vi "test_Read Digital Static In.vi"(8 "error in (no error)":errorcluster, 11 "TestCase in":refnum<class "FPGA Addon Speciality IO Tests.lvclass">) -> (0 "error out":errorcluster, 3 "TestCase out":refnum<class "FPGA Addon Speciality IO Tests.lvclass">)   [LabVIEW 2020, in "FPGA Addon Speciality IO Tests.lvclass"]
uses:
  FPGA Addon Speciality IO Tests.lvclass
  C:/Users/Administrator/Desktop/GIT/niveristand-custom-device-testing-tools/VeriStandTestCase/VeriStandTestCase.lvclass
  <vilib>/addons/_JKI Toolkits/VI Tester/TestCase.llb/TestCase.lvclass
  FPGA Addon Test Class/FPGA Addon Test Class.lvclass
  C:/Program Files (x86)/National Instruments/LabVIEW 2020/vi.lib/addons/_JKI Toolkits/VI Tester/TestCase.llb/TestCase.lvclass
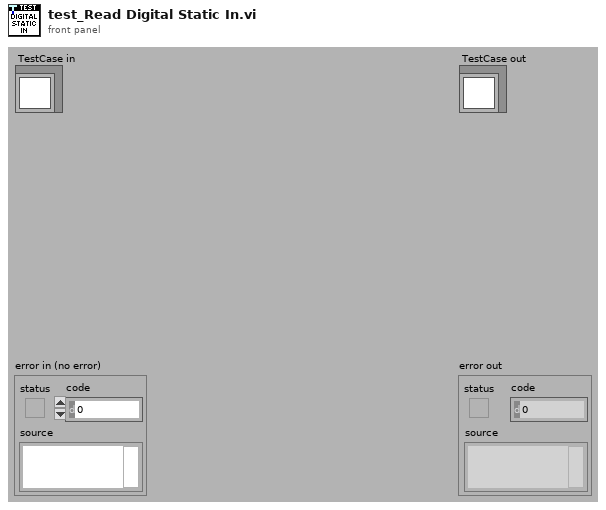
[diagram p1: front panel]
types:
  T1 = typedef "NI_VS Workspace ExecutionAPI.lvlib/WorkspaceAPI.ctl" = refnum<k24>
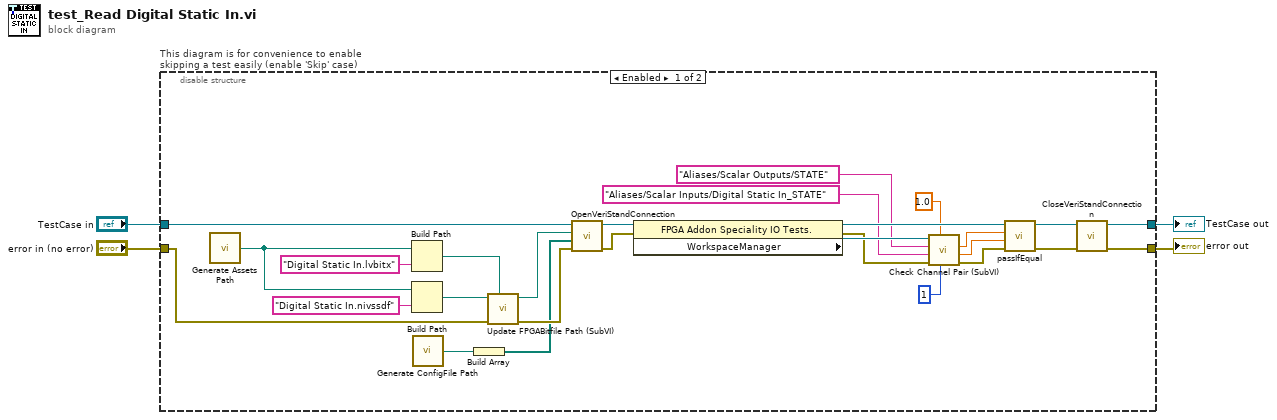
[diagram p0: block diagram]
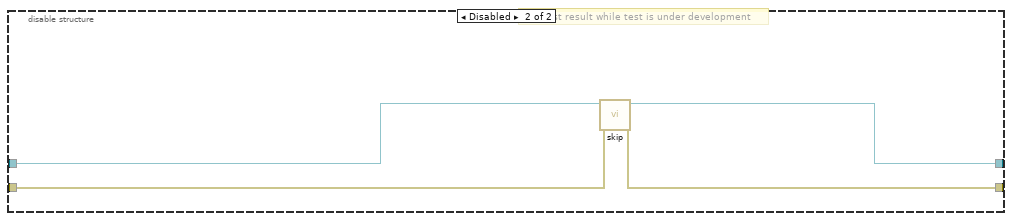
[diagram p2: hidden frame]
diagram:
  n1 = disable-structure "This diagram is for convenience to enable skipping a test easily (enable 'Skip' case)" shown="Enabled" {
    disable-tunnel: "TestCase in" -> [w20 w35]
    disable-tunnel: [w18 w33] -> w1
    disable-tunnel: [w19 w34] -> w3
    disable-tunnel: "error in (no error)" -> [w10 w32]
    frame Enabled {
      n2 = call "Generate Assets Path.vi"() -> ("Assets path"=w13:path)
      n3 = Build Path(base path=w13, name or relative path="Digital Static In.lvbitx") -> (appended path=w14:path)
      n4 = Build Path(base path=w13, name or relative path="Digital Static In.nivssdf") -> (appended path=w15:path)
      n5 = call "Generate ConfigFile Path.vi"() -> ("ConfigFile path"=w12:path)
      n6 = Build Array(w12) -> (w7:path[])
      n7 = call "Update FPGABitfile Path (SubVI).vi"("Bitfile Path"=w14, "error in (no error)"=w10, "System Definition path in"=w15) -> ("error out"=w9:errorcluster, "System Definition path out"=w6:path)  [unwired: 7 in]
      n8 = call-dynamic "OpenVeriStandConnection.vi"("error in (no error)"=w9, "overrides files"=w7, "System Definition File"=w6, "VeriStand Test Case in"=w20) -> ("error out"=w31:errorcluster, "VeriStand Test Case out"=w30:refnum<class "FPGA Addon Speciality IO Tests.lvclass">)  [unwired: 5 in, 1 out]
      n9 = property class="FPGA Addon Speciality IO Tests."(reference=w30, error in=w31) -> (reference out=w29:refnum<class "FPGA Addon Speciality IO Tests.lvclass">, error out=w23:errorcluster, "WorkspaceManager"=w26:T1)
      n10 = call "Check Channel Pair (SubVI).vi"("seconds to wait"=u32 1 ("milliseconds to wait"), "OutputChannel Value in"=1.0 ("Value"), "error in (no error)"=w23, "Input Channel"="Aliases/Scalar Inputs/Digital Static In_STATE" ("Channel"), "Output Channel"="Aliases/Scalar Outputs/STATE" ("Channel"), "WorkspaceManager in"=w26) -> ("error out"=w24:errorcluster, "OutputChannel Value out"=w21:dbl, "InputChanel Value"=w22:dbl)  [unwired: 2 in, 1 out]
      n11 = call-dynamic "passIfEqual.vi"("error in (no error)"=w24, "y"=w21, "x"=w22, "TestCase in"=w29) -> ("error out"=w27:errorcluster, "TestCase out"=w28:refnum<class "FPGA Addon Speciality IO Tests.lvclass">)  [unwired: 6 in]
      n12 = call-dynamic "CloseVeriStandConnection.vi"("error in (no error)"=w27, "VeriStand Test Case in"=w28) -> ("error out"=w19:errorcluster, "VeriStand Test Case out"=w18:refnum<class "FPGA Addon Speciality IO Tests.lvclass">)  [unwired: 8 in]
    }
    frame Disabled {
      # "skip test result while test is under development"
      n13 = call <vilib>:"skip.vi"("error in (no error)"=w32, "TestCase in"=w35) -> ("error out"=w34:errorcluster, "TestCase out"=w33:refnum<class "FPGA Addon Speciality IO Tests.lvclass">)  [unwired: 8 in]
    }
  }
  "error out" <- w3
  "TestCase out" <- w1
